vi "ex4-6.vi"   [LabVIEW 2009]
uses:
  <vilib>/NXT/Block Support/NXT_InputPort.ctl
  <vilib>/NXT/Dual Mode Library/Logging/LogRedData_light.vi
types:
  T1 = cluster{"Sample Time (0.5 sec)":sgl, "Time (10 sec)":sgl}
  T2 = typedef "NXT_InputPort.ctl" = u8
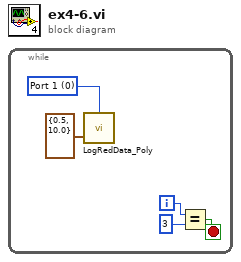
[diagram p0: block diagram]
diagram:
  n1 = while {
    i -> [w3]
    stop <- w2 stop-if-true
    w4 = T2 0 items=["Port 1", "Port 2", "Port 3", "Port 4"] ("Port (Port 3)")
    n2 = call-poly <vilib>:"LogRedData_Poly.vi"("Parameters"=T1 {"Sample Time (0.5 sec)"=0.5, "Time (10 sec)"=10.0}, "Port (Port 3)"=w4) -> ()  [unwired: 2 in, 1 out]
    n3 = Equal?(x=w3, y=3) -> (x = y?=w2:bool)
  }
